vi "Test View Broadcast is Stopped on Clear if Upstreams Error.vi"(8 "error in (no error)":errorcluster, 11 "UI View Test In":refnum<class "View Dev Test.lvclass">) -> (0 "error out":errorcluster, 3 "UI View Test Out":refnum<class "View Dev Test.lvclass">)   [LabVIEW 2020, in "View Dev Test.lvclass"]
uses:
  View Dev Test.lvclass
  View Dev Test.lvclass/View Dev Test.ctl
  source/Framework/View/View.lvclass
  source/Framework/Process/Process.lvclass
  source/Framework/Broadcast Event Helpers/Broadcast Event Helpers.lvlib
  C:/Git/astemes-triarc-framework/source/Framework/Process/Process.lvclass
  C:/Git/astemes-triarc-framework/source/Framework/Base/Base.lvclass
  C:/Git/astemes-triarc-framework/source/Framework/Error Handler Interface/Error Handler Interface.lvclass
  C:/Git/astemes-triarc-framework/source/Framework/Logging/Logging.lvclass
  C:/Git/astemes-triarc-framework/source/Framework/View/View.lvclass
  <vilib>/Astemes/LUnit/Test Case.lvclass
  C:/Git/astemes-triarc-framework/source/Framework Test Suite/Process Test/Process Test.lvclass
  C:/Git/astemes-triarc-framework/source/Framework Test Suite/Base Class Test/Base Test.lvclass
  C:/Program Files (x86)/National Instruments/LabVIEW 2020/vi.lib/Astemes/LUnit/Test Case.lvclass
  C:/Git/astemes-triarc-framework/tests/View Dev Test/View Dev Test.lvclass
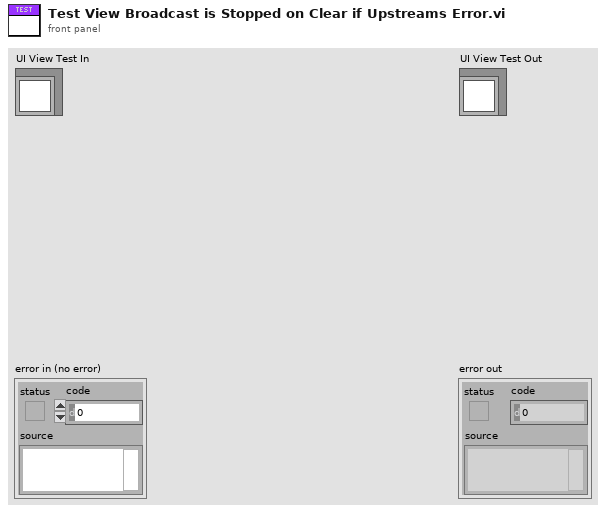
[diagram p1: front panel]
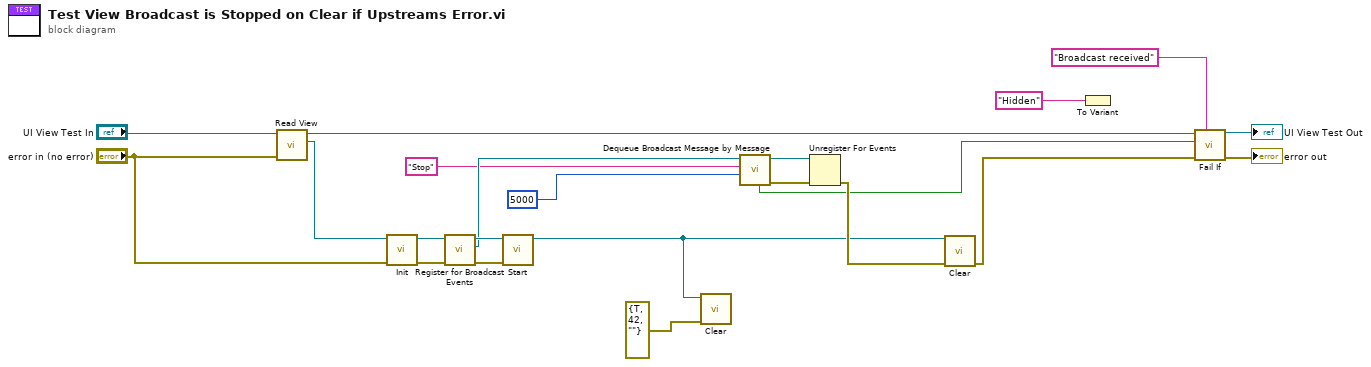
[diagram p0: block diagram]
diagram:
  n1 = call "Read View.vi"("error in (no error)"="error in (no error)", "View Test In"="UI View Test In") -> ("View"=w17:refnum<class "View.lvclass">, "View Test Out"=w20:refnum<class "View Dev Test.lvclass">)  [unwired: 7 in, 1 out]
  n2 = call-dynamic "Init.vi"("error in (no error)"="error in (no error)", "View In"=w17) -> ("error out"=w16:errorcluster, "View Out"=w13:refnum<class "View.lvclass">)  [unwired: 8 in]
  n3 = call "Register for Broadcast Events.vi"("error in (no error)"=w16, "Process In"=w13) -> ("error out"=w14:errorcluster, "Event Registration Refnum Out"=w11:refnum<event-registration>, "Process Out"=w12:refnum<class "View.lvclass">)  [unwired: 7 in]
  n4 = call "Start.vi"("error in (no error)"=w14, "Process In"=w12) -> ("Process Out"=w3:refnum<class "View.lvclass">)  [unwired: 7 in, 2 out]
  n5 = call-dynamic "Clear.vi"("error in (no error)"=errorcluster {"status"=TRUE, "code"=42, "source"=""}, "View In"=w3) -> ()  [unwired: 9 in, 1 out]
  n6 = call "Dequeue Broadcast Message by Message.vi"("Timeout (-1)"=5000, "Message"="Stop", "Event Registration Refnum"=w11) -> ("error out"=w5:errorcluster, "Event Registration Refnum Out"=w8:refnum<event-registration>, "Timed Out?"=w1:bool)  [unwired: 4 in, 2 out]
  n7 = Unregister For Events(event registration refnum=w8, error in=w5) -> (error out=w4:errorcluster)
  n8 = call-dynamic "Clear.vi"("error in (no error)"=w4, "View In"=w3) -> ("error out"=w7:errorcluster)  [unwired: 9 in]
  n9 = To Variant(anything="Hidden") -> ()  [unwired: 1 out]
  n10 = call <vilib>:"Fail If.vi"("Description"="Broadcast received", "error in (no error)"=w7, "Fail?"=w1, "LUnit Test Case In"=w20) -> ("error out"=→"error out":errorcluster, "LUnit Test Case Out"=→"UI View Test Out":refnum<class "View Dev Test.lvclass">)  [unwired: 6 in]
